vi "generator2.vi"() -> ()   [LabVIEW 2025]
panel:
  in  "liczba cykli":i64
  in  "samples":i32=128
  in  "phase":dbl
  in  "Amp":dbl
  out "chart":dbl[](graph)
  in  "stop":bool
  in  "Sygnal":T1(ring)
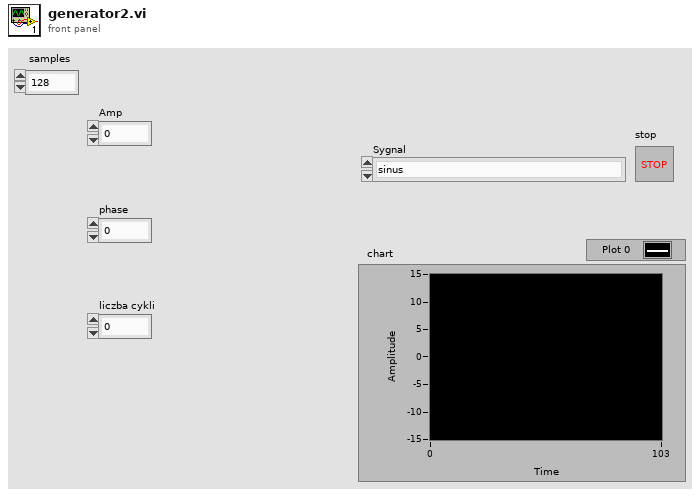
[diagram p1: front panel]
types:
  T1 = enum16{"sinus", "prostokat", "pila", "trojkat", "rozklad losowy", "rozklad normalny"}
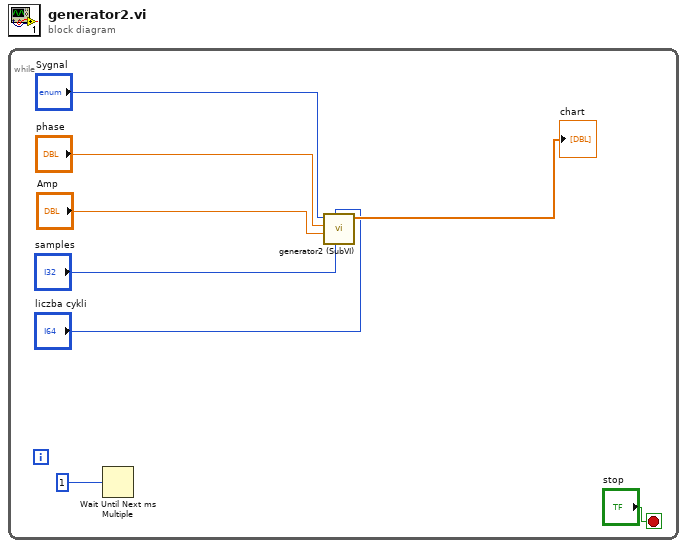
[diagram p0: block diagram]
diagram:
  n1 = while {
    stop <- "stop" stop-if-true
    n2 = Wait Until Next ms Multiple(millisecond multiple=1) -> ()  [unwired: 1 out]
    n3 = call "generator2 (SubVI).vi"("samples"="samples", "liczba cykli"="liczba cykli", "Amp"="Amp", "phase"="phase", "Sygnal"="Sygnal") -> ("Gaussian noise pattern"=→"chart":dbl[])  [unwired: 6 in]
  }
